vi "Get Domain.vi"(11 "Exponential Fit in":refnum<class "Exponential Fit.lvclass">) -> (0 "Xmax":i32, 1 "Xmin":i32, 2 "X range":i32, 3 "Exponential Fit out":refnum<class "Exponential Fit.lvclass">)   [LabVIEW 2013, in "Exponential Fit.lvclass"]
uses:
  Exponential Fit.lvclass
  Exponential Fit.lvclass/Exponential Fit.ctl
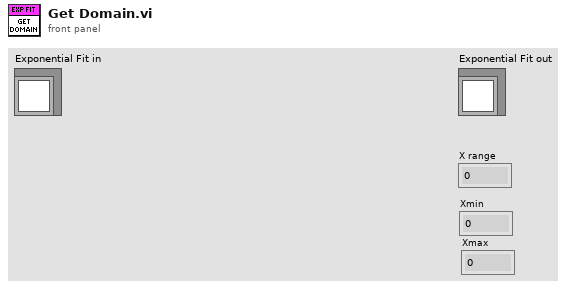
[diagram p1: front panel]
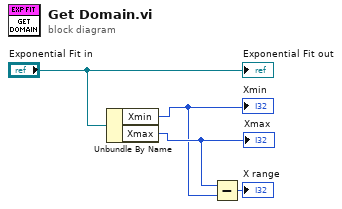
[diagram p0: block diagram]
diagram:
  n1 = Unbundle By Name("Exponential Fit in") -> ("Xmin"=w1:i32, "Xmax"=w2:i32)
  "Xmin" <- w1
  "Xmax" <- w2
  n2 = Subtract(x=w2, y=w1) -> (x-y=→"X range":i32)
  "Exponential Fit out" <- "Exponential Fit in"
